vi "ResetCamera.vi"(8 "error in (no error)":errorcluster, 11 "Game in":refnum<class "Game.lvclass">) -> (0 "error out":errorcluster, 3 "Game out":refnum<class "Game.lvclass">)   [LabVIEW 2019, in "RT_Game.lvlib" / "Game.lvclass"]
uses:
  Game.lvclass
  Engine/MessageCluster.ctl
  Game.lvclass/Game.ctl
  Engine/Engine.lvclass
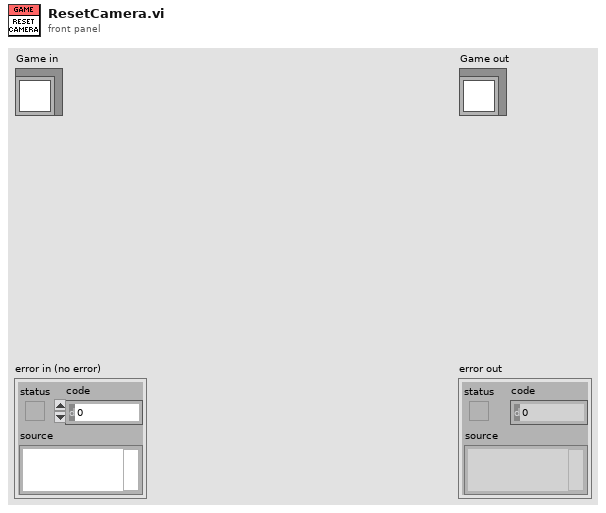
[diagram p1: front panel]
types:
  T1 = typedef "RT_Game.lvlib/Engine.lvclass/MessageCluster.ctl" = cluster{"Message":string, "Data":variant}
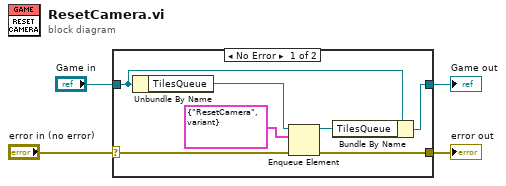
[diagram p0: block diagram]
diagram:
  n1 = case shown="No Error" "error in (no error)" {
    selector: "error in (no error)" -> [w11 w13]
    tunnel: [w8 w13] -> w3
    tunnel: [w10 w12] -> w1
    tunnel: "Game in" -> [w9 w12]
    frame No Error {
      n2 = Unbundle By Name(w9) -> ("TilesQueue"=w7:refnum<queue>)
      n3 = Enqueue Element(queue=w7, element=T1 {"Message"="ResetCamera", "Data"=variant}, error in (no error)=w11) -> (queue out=w6:refnum<queue>, error out=w8:errorcluster)  [unwired: 1 in, 1 out]
      n4 = Bundle By Name(cluster=w9, "TilesQueue"=w6) -> (w10:refnum<class "Game.lvclass">)
    }
    frame Error {
    }
  }
  "error out" <- w3
  "Game out" <- w1
